vi "Sub_Preprocessing_FEA_Mass_Accelerometer.vi"(9 "Element Length":dbl, 10 "accelerometer_mass":dbl, 11 "Matrix w/o BC":dbl[][](array[numeric])) -> (3 "Matrix W/ Accelerometer":dbl[][](array[numeric]))   [LabVIEW 2021]
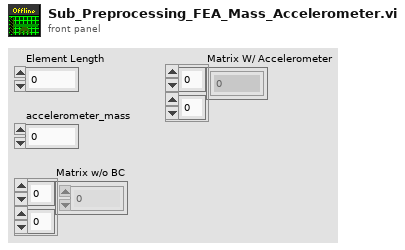
[diagram p1: front panel]
types:
  T1 = cluster{"beam_length":dbl, "youngs_modulus":dbl, "torsion_spring":dbl, "beam_height":dbl, "beam_width":dbl, "beam_density":dbl, "number_of_FEA_nodes":i32, "accelerometer_mass":dbl, "M Matrix":dbl[][], "K Matrix":dbl[][]}
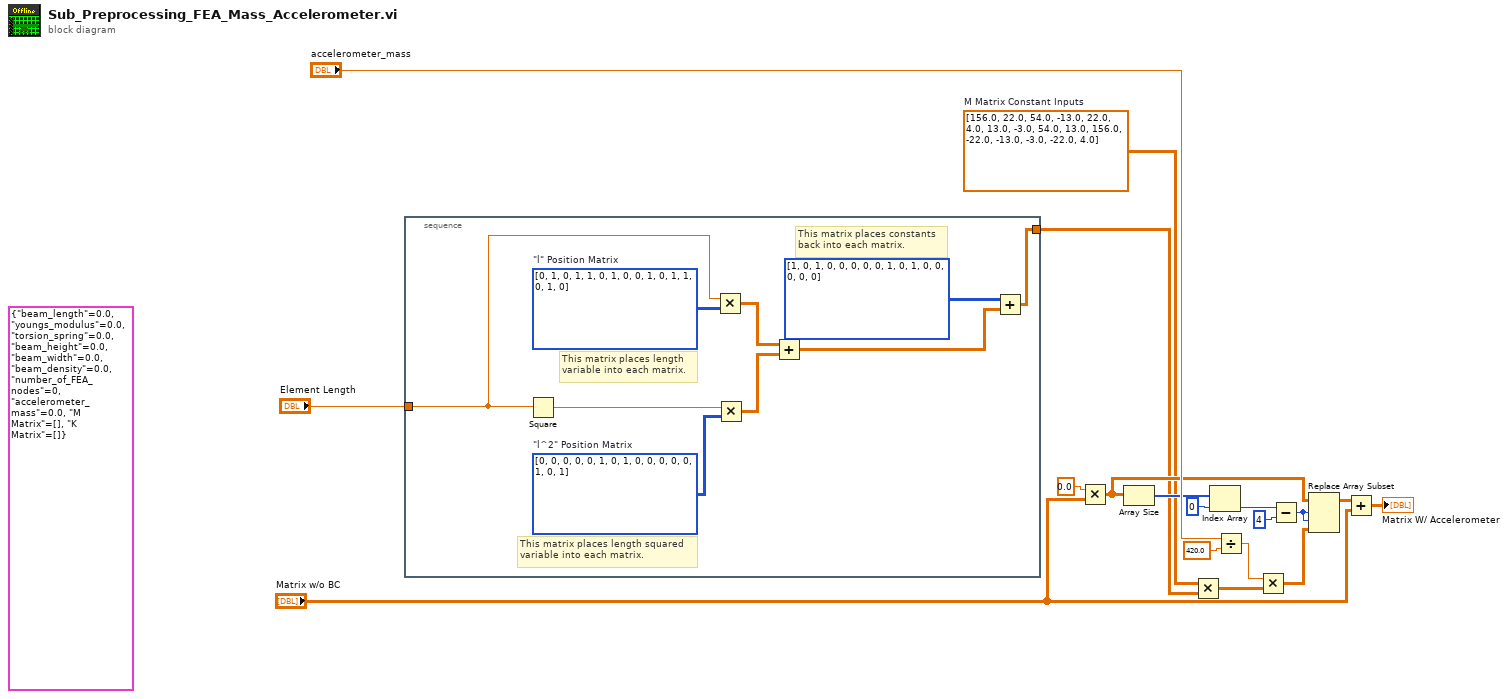
[diagram p0: block diagram]
diagram:
  (unwired) T1 {"beam_length"=0.0, "youngs_modulus"=0.0, "torsion_spring"=0.0, "beam_height"=0.0, "beam_width"=0.0, "beam_density"=0.0, "number_of_FEA_nodes"=0, "accelerometer_mass"=0.0, "M Matrix"=[], "K Matrix"=[]} ("Modeling Parameters")
  w6 = dbl[][] [[156.0, 22.0, 54.0, -13.0], [22.0, 4.0, 13.0, -3.0], [54.0, 13.0, 156.0, -22.0], [-13.0, -3.0, -22.0, 4.0]]  # M Matrix Constant Inputs
  n1 = stacked-sequence {
    tunnel: [w25] -> w8
    tunnel: "Element Length" -> [w27]
    frame #0 {
      w20 = i32[][] [[0, 0, 0, 0], [0, 1, 0, 1], [0, 0, 0, 0], [0, 1, 0, 1]]  # "l^2" Position Matrix
      w19 = i32[][] [[0, 1, 0, 1], [1, 0, 1, 0], [0, 1, 0, 1], [1, 0, 1, 0]]  # "l" Position Matrix
      # "This matrix places length squared\nvariable into each matrix."
      # "This matrix places length \nvariable into each matrix."
      # "This matrix places constants\nback into each matrix."
      n2 = Square(x=w27) -> (x^2=w22:dbl)
      n3 = Multiply(x=w27, y=w19) -> (x*y=w21:dbl[][])
      n4 = Multiply(x=w22, y=w20) -> (x*y=w23:dbl[][])
      n5 = Add(x=w21, y=w23) -> (x+y=w26:dbl[][])
      n6 = Add(x=i32[][] [[1, 0, 1, 0], [0, 0, 0, 0], [1, 0, 1, 0], [0, 0, 0, 0]], y=w26) -> (x+y=w25:dbl[][])
    }
  }
  n7 = Multiply(x=0.0, y="Matrix w/o BC") -> (x*y=w10:dbl[][])
  n8 = Array Size(array=w10) -> (size(s)=w11:i32[])
  n9 = Multiply(x=w6, y=w8) -> (x*y=w5:dbl[][])
  n10 = Index Array(array=w11, index=0) -> (element=w13:i32)
  n11 = Divide(x="accelerometer_mass", y=420.0) -> (x/y=w4:dbl)
  n12 = Multiply(x=w4, y=w5) -> (x*y=w16:dbl[][])
  n13 = Subtract(x=w13, y=4) -> (x-y=w15:i32)
  n14 = Replace Array Subset(array=w10, new element=w16, index (row)=w15, index (col)=w15) -> (w17:dbl[][])
  n15 = Add(x=w17, y="Matrix w/o BC") -> (x+y=→"Matrix W/ Accelerometer":dbl[][])
